vi "NIVS.Waveforms.Group.vi"(8 "error in (no error)":errorcluster, 11 "Cluster":T1) -> (0 "error out":errorcluster)   [LabVIEW 2015, in "Station.Execution.lvlib"]
uses:
  Station.Execution.lvlib
  Types/Main.StateVariables.ctl
  Types/Execute.UserEventRefs.ctl
  <vilib>/NI Veristand/Execution/Workspace/SystemStateRegEventRef.ctl
  <vilib>/NI Veristand/Execution/Workspace/Target State Info.ctl
  <vilib>/NI Veristand/Execution/Workspace/Target State.ctl
  <vilib>/NI Veristand/Execution/WaveformStreaming/Waveform Data Watcher Event Data (DBL).ctl
  <vilib>/NI Veristand/Execution/WaveformStreaming/WaveformStreamSpecification.ctl
  NationalInstruments.VeriStand.ClientAPI
  <vilib>/NI Veristand/Execution/Workspace/SystemStateEventRef.ctl
  <vilib>/NI Veristand/Execution/Workspace/WorkspaceAPI.ctl
  Types/Waveforms.Info.ctl
  <vilib>/NI Veristand/Execution/WaveformStreaming/Registered Waveform Streams Data Event Refnum (DBL).ctl
  <vilib>/NI Veristand/Execution/WaveformStreaming/WaveformDataWatcherDBL.ctl
  <vilib>/NI Veristand/Execution/WaveformStreaming/WaveformStreamingAPI.ctl
  <vilib>/Utility/miscctls.llb/LVPositionTypeDef.ctl
  Types/UI.Object.ctl
  NationalInstruments.VeriStand
  <vilib>/NI Veristand/Execution/Workspace/NI_VS Workspace ExecutionAPI.lvlib
  <vilib>/NI Veristand/Execution/WaveformStreaming/NI_VS Waveform Streaming Interface.lvlib
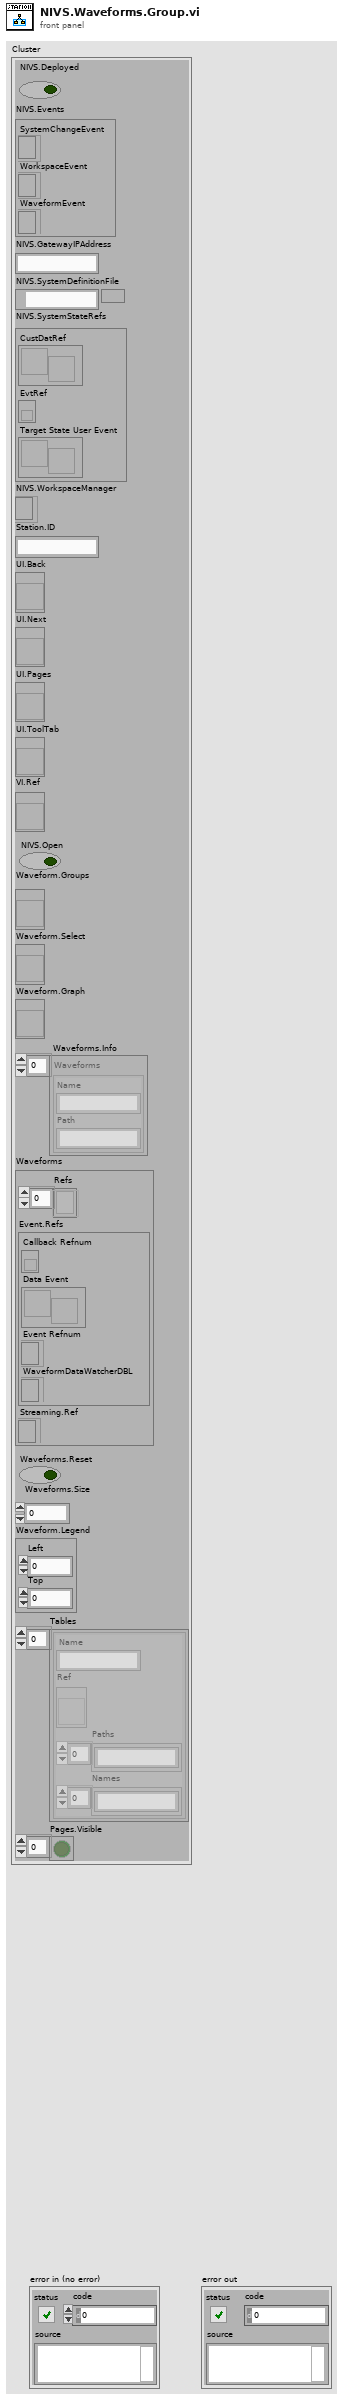
[diagram p1: front panel]
types:
  T1 = typedef "Station.Execution.lvlib/Main.StateVariables.ctl" = cluster{"NIVS.Deployed":bool, "NIVS.Events":T2, "NIVS.GatewayIPAddress":string, "NIVS.SystemDefinitionFile":path, "NIVS.SystemStateRefs":T4, "NIVS.WorkspaceManager":T5, "Station.ID":string, "UI.Back":refnum<vi>, "UI.Next":refnum<vi>, "UI.Pages":refnum<vi>, "UI.ToolTab":refnum<vi>, "VI.Ref":refnum<vi>, "NIVS.Open":bool, "Waveform.Groups":refnum<vi>, "Waveform.Select":refnum<vi>, "Waveform.Graph":refnum<vi>, "Waveforms.Info":T6[], "Waveforms":cluster{"Refs":T7[], "Event.Refs":T8, "Streaming.Ref":T10}, "Waveforms.Reset":bool, "Waveforms.Size":i32, "Waveform.Legend":T11, "Tables":T12[], "Pages.Visible":bool[]}
  T2 = typedef "Station.Execution.lvlib/Execute.UserEventRefs.ctl" = cluster{"SystemChangeEvent":T3, "WorkspaceEvent":refnum<event-registration>, "WaveformEvent":refnum<event-registration>}
  T3 = typedef "NI_VS Workspace ExecutionAPI.lvlib/SystemStateRegEventRef.ctl" = refnum<event-registration>
  T4 = typedef "NI_VS Workspace ExecutionAPI.lvlib/SystemStateEventRef.ctl" = cluster{"CustDatRef":refnum<user-event>, "EvtRef":refnum<k27>, "Target State User Event":refnum<user-event>}
  T5 = typedef "NI_VS Workspace ExecutionAPI.lvlib/WorkspaceAPI.ctl" = refnum<k24>
  T6 = typedef "Station.Execution.lvlib/Waveforms.Info.ctl" = cluster{"Name":string, "Path":string}
  T7 = typedef "NI_VS Waveform Streaming Interface.lvlib/WaveformStreamSpecification.ctl" = refnum<k24>
  T8 = typedef "NI_VS Waveform Streaming Interface.lvlib/Registered Waveform Streams Data Event Refnum (DBL).ctl" = cluster{"Callback Refnum":refnum<k27>, "Data Event":refnum<user-event>, "Event Refnum":refnum<event-registration>, "WaveformDataWatcherDBL":T9}
  T9 = typedef "NI_VS Waveform Streaming Interface.lvlib/WaveformDataWatcherDBL.ctl" = refnum<k24>
  T10 = typedef "NI_VS Waveform Streaming Interface.lvlib/WaveformStreamingAPI.ctl" = refnum<k24>
  T11 = typedef "LVPositionTypeDef.ctl" = cluster{"Left":i32, "Top":i32}
  T12 = typedef "Station.Execution.lvlib/UI.Object.ctl" = cluster{"Name":string, "Ref":refnum<vi>, "Paths":string[], "Names":string[]}
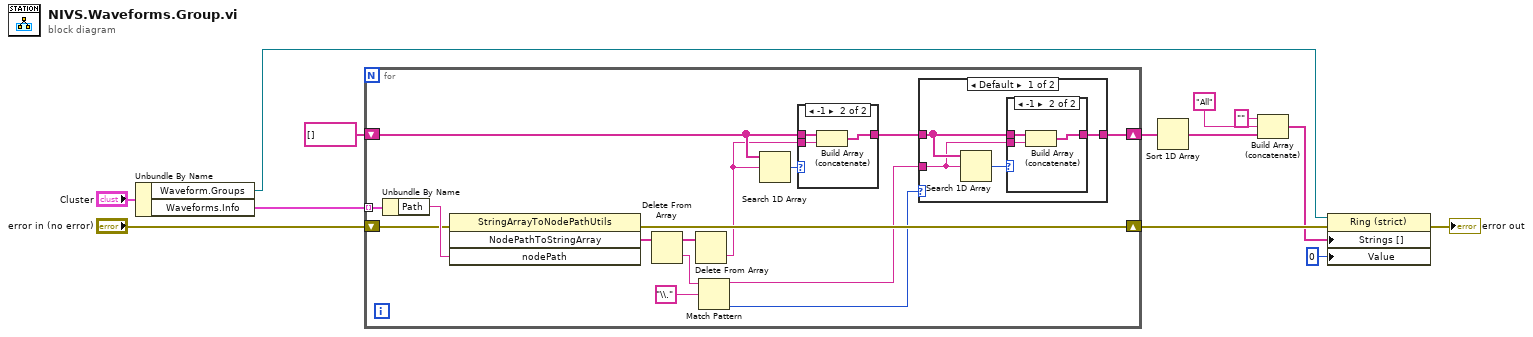
[diagram p0: block diagram]
diagram:
  n1 = Unbundle By Name("Cluster") -> ("Waveform.Groups"=w7:refnum<vi>, "Waveforms.Info"=w11:T6[])
  n2 = for {
    tunnel: w11 -> [w28] mode=indexing
    shift-right: [w25] -> w9
    shift-left: "error in (no error)" -> [w26]
    shift-right: [w16] -> w6
    shift-left: string[] [] -> [w21]
    n3 = Unbundle By Name(w28) -> ("Path"=w27:string)
    n4 = invoke class="StringArrayToNodePathUtils" method="NodePathToStringArray"(error in=w26, "nodePath"=w27) -> (error out=w25:errorcluster, "NodePathToStringArray"=w24:string[])  [unwired: 2 in, 2 out]
    n5 = Delete From Array(array=w24) -> (deleted portion=w19:string, array with subset deleted=w23:string[])  [unwired: 2 in]
    n6 = Delete From Array(array=w23) -> (deleted portion=w20:string)  [unwired: 2 in, 1 out]
    n7 = Match Pattern(string=w19, regular expression="\\.") -> (before substring=w14:string, offset past match=w17:i32)  [unwired: 1 in, 2 out]
    n8 = Search 1D Array(1D array=w21, element=w20) -> (index of element=w22:i32)  [unwired: 1 in]
    n9 = case shown="-1" w22 {
      tunnel: w21 -> [w38 w41]
      tunnel: w20 -> [_ w40]
      tunnel: [w38 w39] -> w15
      frame Default {
      }
      frame -1 {
        n10 = Build Array (concatenate)(w41, w40) -> (w39:string[])
      }
    }
    n11 = case shown="Default" w17 {
      tunnel: w15 -> [w31 w37]
      tunnel: [w29 w37] -> w16
      tunnel: w14 -> [w30 _]
      frame Default {
        n12 = Search 1D Array(1D array=w31, element=w30) -> (index of element=w32:i32)  [unwired: 1 in]
        n13 = case shown="-1" w32 {
          tunnel: w31 -> [w33 w36]
          tunnel: w30 -> [_ w35]
          tunnel: [w33 w34] -> w29
          frame Default {
          }
          frame -1 {
            n14 = Build Array (concatenate)(w36, w35) -> (w34:string[])
          }
        }
      }
      frame -1 {
      }
    }
  }
  n15 = Sort 1D Array(array=w6) -> (sorted array=w3:string[])
  n16 = Build Array (concatenate)("" ("element"), "All", w3) -> (w4:string[])
  n17 = property class="Ring (strict)"(reference=w7, error in=w9, "Strings []"=w4, "Value"=u8 0) -> (error out=→"error out":errorcluster)  [unwired: 1 out]
